vi "Anemo Receiver with Threshold.vi"() -> ()   [LabVIEW 2011]
doc: "Use this VI with the UDP Sender VI. Run this VI first.\n\nThe UDP protocol differs from TCP in that there is no error-checking with the packets of information that are sent, and thus no guarantee whatsoever that an intended recipient will actually receive a given piece of data.\n\nUDP does offer the ability to \"broadcast\" data across a network--simply specify an IP Address of all ones (255.255.255.255) to attempt to broadcast information network-wide. Keep in mind that routers and other network hardware will generally refuse to forward the broadcast beyond certain points, so the extent of the broadcast will in practice be limited."
uses:
  <vilib>/Utility/file.llb/Write To Spreadsheet File (string).vi
  Anemometry/Anemometry Sub Vis/Globals/Meas_global.vi
panel:
  out "Boolean":bool
  in  "Threshold":dbl=9.0
  out "output 3":dbl
  out "output 2":dbl
  out "resulting string":string
  out "data out 3":string
  in  "Port 2":u16=61557
  out "data out":string
  in  "max bytes/read":i32=548
  in  "Port":u16=61558
  in  "stop":bool
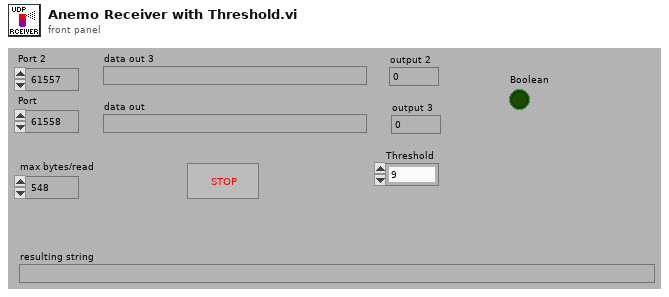
[diagram p1: front panel]
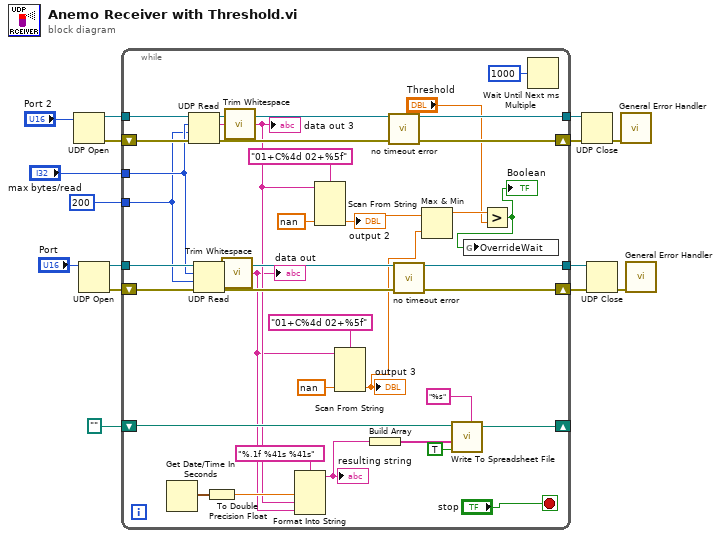
[diagram p0: block diagram]
diagram:
  n1 = UDP Open(11:"Port 2") -> (port=w4:refnum<k16>, 0:w3:errorcluster)  [unwired: 4 in, 1 out]
  n2 = UDP Open(11:"Port") -> (port=w13:refnum<k16>, 0:w14:errorcluster)  [unwired: 4 in, 1 out]
  n3 = while {
    tunnel: [w49] -> w12
    tunnel: w13 -> [w50]
    shift-left: w14 -> [w51]
    shift-right: [w47] -> w11
    tunnel: "max bytes/read" -> [w39]
    tunnel: 200 -> [w38]
    tunnel: [w42] -> w5
    tunnel: w4 -> [w41]
    shift-right: [w44] -> w6
    shift-left: w3 -> [w40]
    shift-right: [w32] -> _
    shift-left: path "" -> [w28]
    stop <- "stop" stop-if-true
    n4 = Get Date/Time In Seconds() -> (seconds since 1Jan1904=w37:timestamp)
    n5 = UDP Read(connection ID=w41, max size (548)=w39, timeout ms (25000)=w38, 8:w40) -> (data out=w34:string, error out=w43:errorcluster, 3:w42:refnum<k16>)  [unwired: 2 out]
    n6 = UDP Read(connection ID=w50, max size (548)=w39, timeout ms (25000)=w38, 8:w51) -> (data out=w35:string, error out=w48:errorcluster, 3:w49:refnum<k16>)  [unwired: 2 out]
    n7 = To Double Precision Float(number=w37) -> (double precision float=w36:dbl)
    n8 = call <vilib>:"Trim Whitespace.vi"("string"=w35) -> ("trimmed string"=w21:string)  [unwired: 1 in]
    "data out" <- w21
    n9 = call <vilib>:"Trim Whitespace.vi"("string"=w34) -> ("trimmed string"=w26:string)  [unwired: 1 in]
    "data out 3" <- w26
    n10 = Format Into String(format string="%.1f %41s %41s", w36, w26, w21) -> (resulting string=w31:string)  [unwired: 2 in, 1 out]
    "resulting string" <- w31
    n11 = Scan From String(format string="01+C%4d 02+%5f", input string=w26, default 2=nan ("default value 2")) -> (output 2=w20:dbl)  [unwired: 4 in, 3 out]
    "output 2" <- w20
    n12 = Scan From String(format string="01+C%4d 02+%5f", input string=w21, default 2=nan ("default value 2")) -> (output 2=w19:dbl)  [unwired: 4 in, 3 out]
    "output 3" <- w19
    n13 = Build Array(w31) -> (w29:string[])
    n14 = call "no timeout error.vi"("error in (no error)"=w43) -> ("error out"=w44:errorcluster)
    n15 = call "no timeout error.vi"("error in (no error)"=w48) -> ("error out"=w47:errorcluster)
    n16 = Max & Min(x=w20, y=w19) -> (max(x,y)=w18:dbl)  [unwired: 1 out]
    n17 = call-poly <vilib>:"Write To Spreadsheet File.vi"("format (%s)"="%s" ("format (%.3f)"), "append to file? (new file:F)"=TRUE, "1D data"=w29, "file path (dialog if empty)"=w28) -> ("new file path (Not A Path if cancelled)"=w32:path)  [unwired: 4 in]
    n18 = Greater?(x=w18, y="Threshold") -> (0:w16:bool)
    "Boolean" <- w16
    n19 = global write "Meas_global.vi" "OverrideWait"(w16) -> ()
    n20 = Wait Until Next ms Multiple(millisecond multiple=u32 1000) -> ()  [unwired: 1 out]
  }
  n21 = UDP Close(connection ID=w5, 8:w6) -> (error out=w7:errorcluster)  [unwired: 1 out]
  n22 = UDP Close(connection ID=w12, 8:w11) -> (error out=w10:errorcluster)  [unwired: 1 out]
  n23 = call <vilib>:"General Error Handler.vi"("error in (no error)"=w7) -> ()  [unwired: 10 in, 5 out]
  n24 = call <vilib>:"General Error Handler.vi"("error in (no error)"=w10) -> ()  [unwired: 10 in, 5 out]
